vi "Test Coffee Shop Add Barista.vi"(8 "error in (no error)":errorcluster, 11 "Coffee Shop Test In":refnum<class "Coffee Shop Test.lvclass">) -> (0 "error out":errorcluster, 3 "Coffee Shop Test Out":refnum<class "Coffee Shop Test.lvclass">)   [LabVIEW 2020, in "Coffee Shop Test.lvclass"]
uses:
  Coffee Shop Test.lvclass
  C:/Program Files (x86)/National Instruments/LabVIEW 2020/vi.lib/Asteme/LUnit/Test Case.lvclass
  Processes/Coffee Shop/Coffee Shop.lvclass
  C:/Program Files (x86)/National Instruments/LabVIEW 2020/vi.lib/Asteme/Triarc Framework/Process/Process.lvclass
  C:/Program Files (x86)/National Instruments/LabVIEW 2020/vi.lib/Asteme/Triarc Framework/Application/Application.lvclass
  <vilib>/Asteme/Triarc Framework/Process/Process.lvclass/Process.ctl
  <vilib>/Asteme/Triarc Framework/Application/Application.lvclass/Application.ctl
  <vilib>/Asteme/LUnit/Test Case.lvclass/Test Case.ctl
  <vilib>/Asteme/LUnit/LUnit Assertion Result.lvclass/LUnit Assertion Result.ctl
  <vilib>/Asteme/Triarc Framework/Process/Public/Lifecycle/Get Lifecycle State.vi
  <vilib>/Asteme/Triarc Framework/Process/Protected/Messaging/Request Message.vi
  <vilib>/Asteme/Triarc Framework/Process/Private/SubVIs/Wait for finish.vi
  <vilib>/Asteme/Triarc Framework/Process/Protected/Messaging/Enqueue Message.vi
  <vilib>/Asteme/Triarc Framework/Process/Private/SubVIs/Set Lifecycle State.vi
  <vilib>/Asteme/LUnit/Palette/Pass.vi
  <vilib>/Asteme/LUnit/Palette/Fail.vi
  <vilib>/Asteme/LUnit/Variant to string.vi
  <vilib>/Asteme/LUnit/Set Assertion Type.vi
  <vilib>/Utility/error.llb/Clear Errors.vi
  <vilib>/Asteme/Triarc Framework/Process/Private/SubVIs/Enqueue Request Message.vi
  <vilib>/AdvancedString/1D String Array to Delimited String.vi
  <vilib>/Asteme/LUnit/Add test result.vi
  <vilib>/Asteme/LUnit/LUnit Write Passed.vi
  <vilib>/Asteme/LUnit/LUnit Get Test Case.vi
  <vilib>/Asteme/LUnit/Assertion Result/LUnit Get Test Name.vi
  <vilib>/Asteme/LUnit/LUnit Write Message.vi
  <vilib>/Asteme/LUnit/LUnit Write Description.vi
  <vilib>/Asteme/LUnit/LUnit Write Assertion Type.vi
  <vilib>/Asteme/LUnit/Read Test Case Name.vi
  <vilib>/Asteme/Triarc Framework/Application/Application.lvclass
  <vilib>/Utility/error.llb/Error Cluster From Error Code.vi
  <vilib>/Asteme/Triarc Framework/Process/Private/SubVIs/Wait for Response Message.vi
  <vilib>/Utility/Data Type/Get Type Information.vi
  <vilib>/Utility/LVClass/Get LV Class Name.vi
  <vilib>/Asteme/Triarc Framework/Process/Process.lvclass
  <vilib>/Asteme/LUnit/LUnit Assertion Result.lvclass
  <vilib>/Asteme/LUnit/Test Case.lvclass
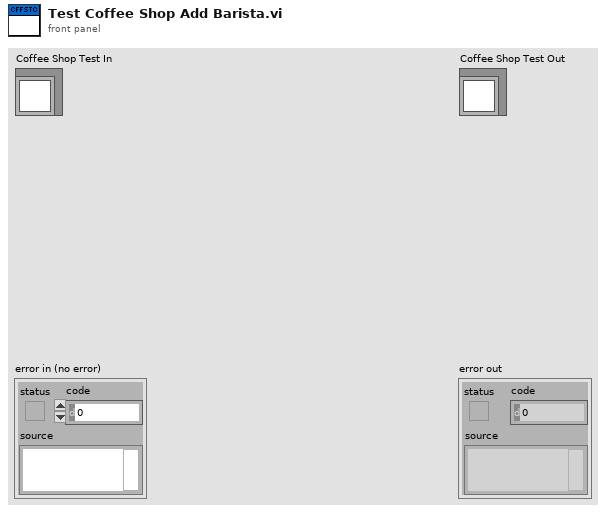
[diagram p1: front panel]
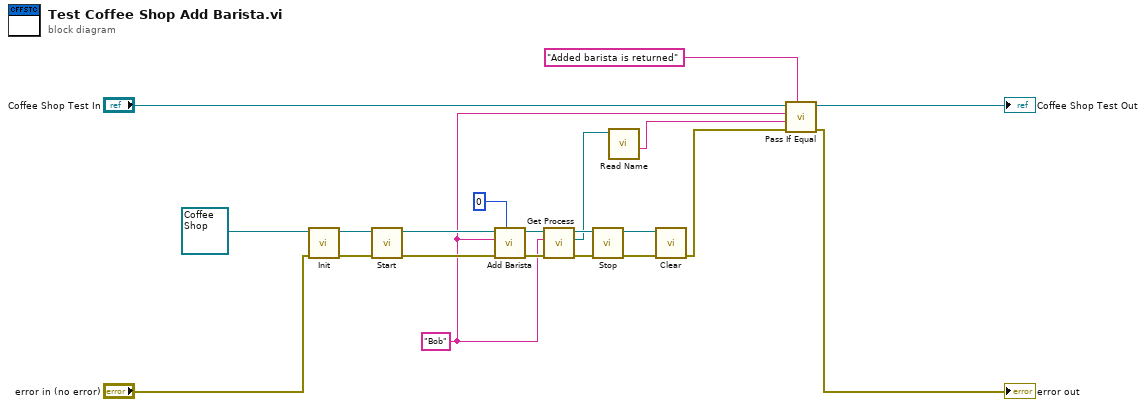
[diagram p0: block diagram]
diagram:
  w4 = "Bob" ("Name")
  n1 = call-dynamic "Init.vi"("error in (no error)"="error in (no error)", "Process In"=refnum<class "Coffee Shop.lvclass"> refnum ("Coffee Shop.lvclass")) -> ("error out"=w19:errorcluster, "Process Out"=w20:refnum<class "Coffee Shop.lvclass">)  [unwired: 8 in]
  n2 = call <vilib>:"Start.vi"("error in (no error)"=w19, "Process In"=w20) -> ("error out"=w14:errorcluster, "Process Out"=w13:refnum<class "Coffee Shop.lvclass">)  [unwired: 8 in]
  n3 = call "Add Barista.vi"("Time Scale [ms]"=u32 0, "error in (no error)"=w14, "Name"=w4, "Coffee Shop in"=w13) -> ("error out"=w15:errorcluster, "Coffee Shop out"=w6:refnum<class "Coffee Shop.lvclass">)  [unwired: 6 in]
  n4 = call <vilib>:"Get Process.vi"("error in (no error)"=w15, "Process Name"=w4, "Rig In"=w6) -> ("error out"=w7:errorcluster, "App Process"=w3:refnum<class "Process.lvclass">, "Rig Out"=w5:refnum<class "Coffee Shop.lvclass">)  [unwired: 6 in]
  n5 = call <vilib>:"Stop.vi"("error in (no error)"=w7, "Process In"=w5) -> ("error out"=w17:errorcluster, "Process Out"=w18:refnum<class "Coffee Shop.lvclass">)  [unwired: 7 in, 1 out]
  n6 = call-dynamic "Read Name.vi"("Process In"=w3) -> ("Name"=w2:string)  [unwired: 7 in, 3 out]
  n7 = call-dynamic "Clear.vi"("error in (no error)"=w17, "Application In"=w18) -> ("error out"=w10:errorcluster)  [unwired: 9 in]
  n8 = call <vilib>:"Pass If Equal.vi"("Description"="Added barista is returned", "error in (no error)"=w10, "Actual"=w2, "Expected"=w4, "Test Case In"="Coffee Shop Test In") -> ("error out"=→"error out":errorcluster, "Test Case Out"=→"Coffee Shop Test Out":refnum<class "Coffee Shop Test.lvclass">)  [unwired: 5 in]
